vi "to string.vi"(8 "error in":errorcluster, 11 "EthernetIP configuration in":refnum<class "EIP Tags Configuration.lvclass">) -> (0 "error out":errorcluster, 1 "data":string, 2 "version":string, 3 "EthernetIP configuration out":refnum<class "EIP Tags Configuration.lvclass">)   [LabVIEW 2013, in "EIP Tags Configuration.lvclass"]
doc: "Provides an interface for saving a module configuration to a file or other serialized data source. It is recommended that all children of this class store data in two sets--data required for its own initialization, and any data required for parent initialization--and that each implementation uses the <b>Call Parent Method</b> primitive to serialize parent information."
uses:
  EIP Tags Configuration.lvclass
  <vilib>/NI/Tag Bus Module Framework/module configuration/TBM module configuration.lvclass
  EIP Tags Configuration.lvclass/EIP Tags Configuration.ctl
  channel/EIP Tags Channel.lvclass
  <vilib>/NI/Configuration Framework/serializable configuration/NISE_CEF_serializable configuration.lvclass
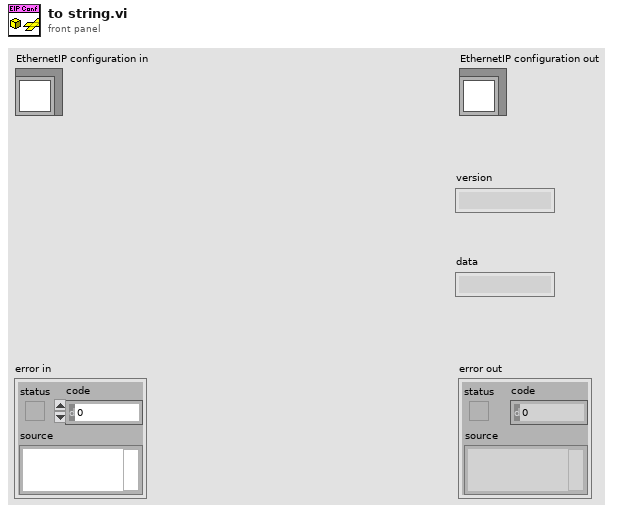
[diagram p1: front panel]
types:
  T1 = typedef "EIP Tags Configuration.lvclass/eip tag definition.ctl" = cluster{"eip tag types":T2, "unique tag name":string, "Number of Elements":u32}
  T2 = typedef "EIP Tags Configuration.lvclass/eip tag types.ctl" = enum16{"SINT", "INT", "DINT", "REAL", "BOOL", "STRING"}
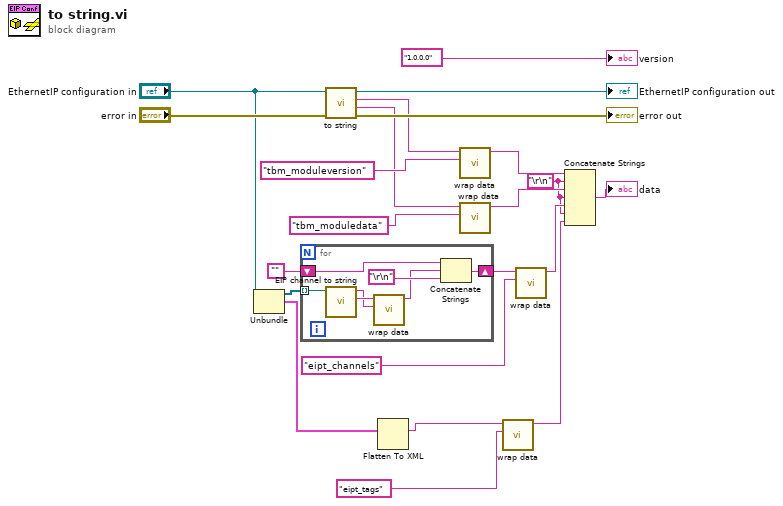
[diagram p0: block diagram]
diagram:
  w6 = "\r\n"
  n1 = Unbundle("EthernetIP configuration in") -> (w9:refnum<class "EIP Tags Channel.lvclass">[], w3:T1[])  [unwired: 1 out]
  n2 = for {
    tunnel: w9 -> [w29] mode=indexing
    shift-right: [w25] -> w7
    shift-left: "" -> [w24]
    n3 = call "EIP channel to string.vi"("channel in"=w29) -> ("channel data"=w28:string, "identifier"=w27:string)  [unwired: 9 in]
    n4 = call <vilib>:"wrap data.vi"("identifier"=w27, "data to wrap"=w28) -> ("wrapped data"=w23:string)  [unwired: 9 in]
    n5 = Concatenate Strings(w24, w23, "\r\n") -> (w25:string)
  }
  n6 = call-parent "to string.vi"("error in"="error in", "module configuration in"="EthernetIP configuration in") -> ("error out"=→"error out":errorcluster, "data"=w14:string, "version"=w15:string, "module configuration out"=→"EthernetIP configuration out":refnum<class "EIP Tags Configuration.lvclass">)  [unwired: 6 in]
  n7 = Flatten To XML(anything=w3) -> (xml string=w2:string)
  n8 = call <vilib>:"wrap data.vi"("identifier"="tbm_moduleversion" ("additional identifier"), "data to wrap"=w15) -> ("wrapped data"=w17:string)  [unwired: 9 in]
  n9 = call <vilib>:"wrap data.vi"("identifier"="tbm_moduledata" ("additional identifier"), "data to wrap"=w14) -> ("wrapped data"=w16:string)  [unwired: 9 in]
  n10 = call <vilib>:"wrap data.vi"("identifier"="eipt_tags" ("additional identifier"), "data to wrap"=w2) -> ("wrapped data"=w4:string)  [unwired: 9 in]
  n11 = call <vilib>:"wrap data.vi"("identifier"="eipt_channels" ("additional identifier"), "data to wrap"=w7) -> ("wrapped data"=w11:string)  [unwired: 9 in]
  n12 = Concatenate Strings(w17, w6, w16, w6, w11, w6, w4) -> (→"data":string)
  "version" <- "1.0.0.0" ("current version")
